vi "Stop Core.vi"(10 "final error code":i32, 11 "Admin_Actor in":refnum<class "Admin_Actor.lvclass">) -> (3 "Admin_Actor out":refnum<class "Admin_Actor.lvclass">)   [LabVIEW 2015, in "Admin_Actor.lvlib" / "Admin_Actor.lvclass"]
doc: "(<B>Filename</B>: Actor Framework.lvlib:Actor.lvclass:Stop Core.vi)\n\nDefines what the actor does before it stops. Use the <B>final error code</B> input to determine whether the actor shut down in response to an error.\n\nBy default, this method does nothing. A descendant class may override it to define behavior, such as shutting down any processes the actor initiated in its override of the Actor Core method."
uses:
  Admin_Actor.lvclass
  User_Actor/User_Actor/User_Actor.lvclass
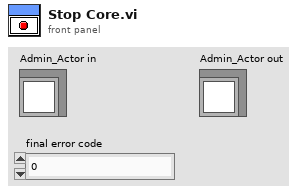
[diagram p1: front panel]
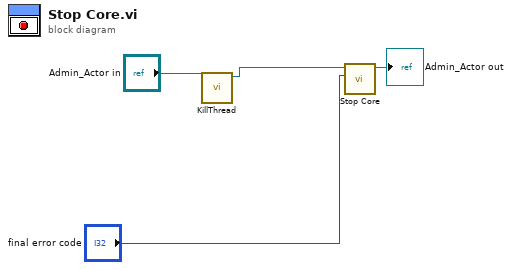
[diagram p0: block diagram]
diagram:
  n1 = call "KillThread.vi"("Admin_Actor in"="Admin_Actor in") -> ("Admin_Actor out"=w1:refnum<class "Admin_Actor.lvclass">)  [unwired: 9 in, 1 out]
  n2 = call-parent "Stop Core.vi"("final error code"="final error code", "Actor in"=w1) -> ("Actor out"=→"Admin_Actor out":refnum<class "Admin_Actor.lvclass">)  [unwired: 9 in]
